vi "Store Multicarrier Custom CDMA State.vi"(0 "VISA Resource Name":refnum<visa-resource-name>, 5 "File Name (CDMA_DATA)":string="CDMA_DATA", 11 "error in (no error)":errorcluster {"code" format="%.0x"}) -> (4 "VISA Resource Name Out":refnum<visa-resource-name>, 15 "error out":errorcluster {"code" format="%.0x"})   [LabVIEW 2012, in "Agilent ESG Series.lvlib"]
doc: "This VI is used to store the current multicarrier setup information.\nAfterward, you can recall this custom state from the instrument's memory with the Config CDMA.vi. - CDMA Select - MULTICARRIER and Multicarrier - CUSTOM\n\nThe stored file contains information including the digital modulation format, number of carriers, frequency spacing, and power settings for the multicarrier setup. \n\nThis VI is valid only on instruments with the UND and UN5 options or on instrument E4438C with option 401."
uses:
  <instrlib>/Agilent ESG Series/Agilent ESG Series.lvlib
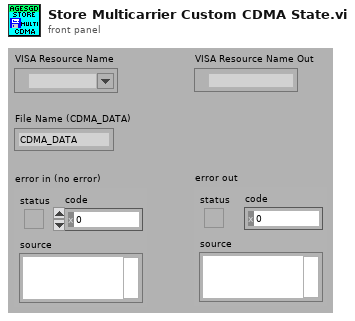
[diagram p1: front panel]
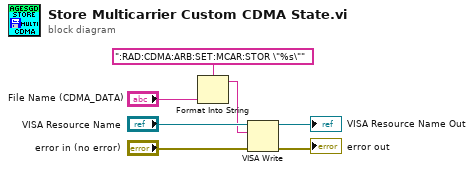
[diagram p0: block diagram]
diagram:
  n1 = Format Into String(format string=":RAD:CDMA:ARB:SET:MCAR:STOR \"%s\"", "File Name (CDMA_DATA)") -> (resulting string=w5:string)  [unwired: 2 in, 1 out]
  n2 = VISA Write(VISA resource name="VISA Resource Name", write buffer=w5, error in (no error)="error in (no error)") -> (VISA resource name out=→"VISA Resource Name Out":refnum<visa-resource-name>, error out=→"error out":errorcluster)  [unwired: 1 out]
